vi "MICSD Do CCA.vi"(8 "error in (no error)":errorcluster, 9 "Use Averaging?":bool=TRUE, 10 "RSSI Mode":u8, 11 "VISA Resource Name":refnum<visa-resource-name>) -> (0 "error out":errorcluster, 1 "CCA Data":u16[](array[numeric]) format="%04x", 2 "Selected Channel":u8, 3 "dup VISA Resource Name":refnum<visa-resource-name>)   [LabVIEW 2020]
uses:
  <vilib>/Instr/_visa.llb/VISA Configure Serial Port (Instr).vi
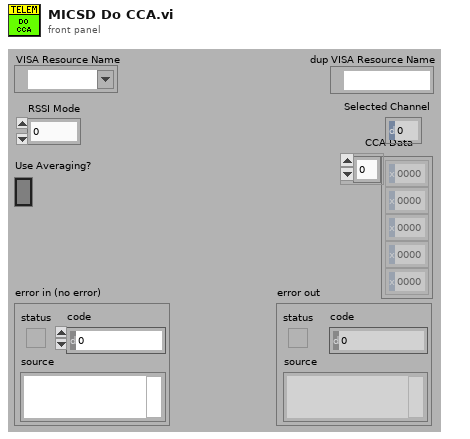
[diagram p1: front panel]
types:
  T1 = cluster{"Command Token":u8, "Length":u16, "Pack Data":u8[]}
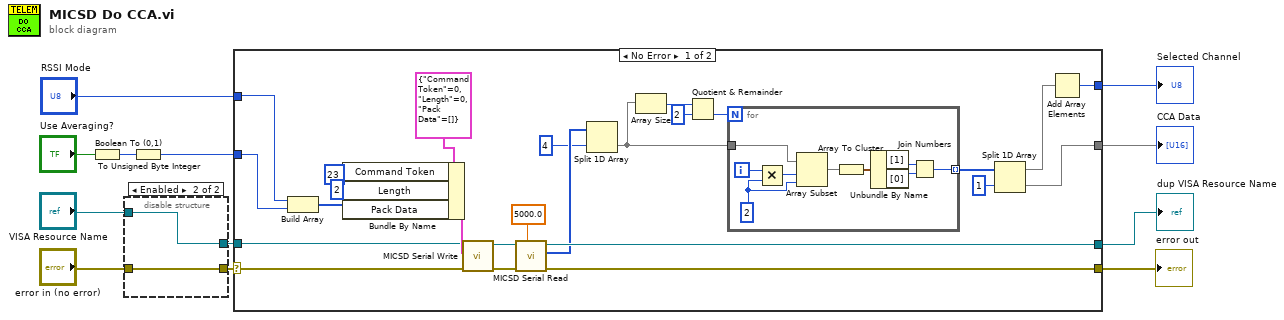
[diagram p0: block diagram]
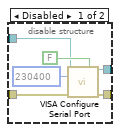
[diagram p2: hidden frame]
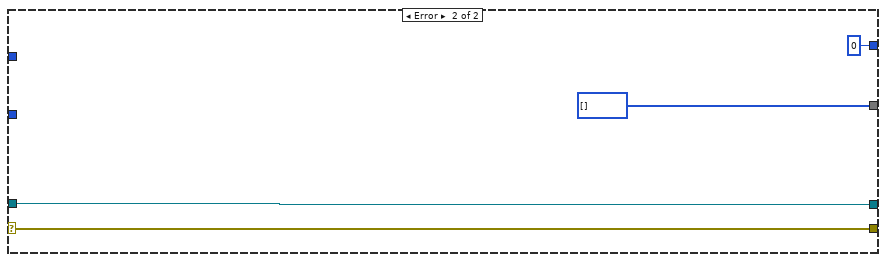
[diagram p3: hidden frame]
diagram:
  n1 = Boolean To (0,1)(Boolean="Use Averaging?") -> (0, 1=w3:i16)
  n2 = disable-structure shown="Enabled" {
    disable-tunnel: [w16 w19] -> w12
    disable-tunnel: [w15 w20] -> w11
    disable-tunnel: "VISA Resource Name" -> [w14 w20]
    disable-tunnel: "error in (no error)" -> [w13 w19]
    frame Disabled {
      n3 = call-poly "VISA Configure Serial Port"("VISA resource name"=w14, "Enable Termination\nChar (T)"=FALSE ("Enable Termination\nChar (T)"), "baud rate (9600)"=u32 230400, "error in (no error)"=w13) -> ("VISA resource name out"=w15:refnum<visa-resource-name>, "error out"=w16:errorcluster)  [unwired: 10 in]
    }
    frame Enabled {
    }
  }
  n4 = To Unsigned Byte Integer(number=w3) -> (unsigned 8bit integer=w2:u8)
  n5 = case shown="No Error" w12 {
    selector: w12 -> [w33 w58]
    tunnel: [w40 w58] -> w7
    tunnel: w11 -> [w34 w57]
    tunnel: [w39 w57] -> w8
    tunnel: [w24 u8[] []] -> w6
    tunnel: "RSSI Mode" -> [w31 _]
    tunnel: w2 -> [w30 _]
    tunnel: [w22 u16 0] -> w1
    frame No Error {
      n6 = Build Array(w31, w30) -> (w32:u8[])
      n7 = Bundle By Name(cluster=T1 {"Command Token"=0, "Length"=0, "Pack Data"=[]} ("Write Data"), "Command Token"=u8 23, "Length"=u16 2, "Pack Data"=w32) -> (w45:T1)
      n8 = call "MICSD Serial Write.vi"("error in (no error)"=w33, "Write Data"=w45, "VISA Resource Name"=w34) -> ("error out"=w38:errorcluster, "DUP Visa Resource Name"=w43:refnum<visa-resource-name>)  [unwired: 7 in]
      n9 = call "MICSD Serial Read.vi"("Timeout(mS)"=5000.0, "error in (no error)"=w38, "VISA Resource Name"=w43) -> ("error out"=w40:errorcluster, "Read Data"=w37:u8[], "DUP Visa Resource Name"=w39:refnum<visa-resource-name>)  [unwired: 6 in]
      n10 = Split 1D Array(array=w37, index=4) -> (second subarray=w29:u8[])  [unwired: 1 out]
      n11 = Array Size(array=w29) -> (size(s)=w28:i32)
      n12 = Quotient & Remainder(x=w28, y=2) -> (floor(x/y)=w27:i32)  [unwired: 1 out]
      n13 = for {
        N: w27 -> [_]
        tunnel: w29 -> [w51]
        tunnel: [w46] -> w25 mode=indexing
        i -> [w54]
        w52 = 2 ("y")
        n14 = Multiply(x=w54, y=w52) -> (x*y=w53:i32)
        n15 = Array Subset(array=w51, index=w53, length=w52) -> (w50:u8[])
        n16 = Array To Cluster(array=w50) -> (cluster=w49:cluster{"[0]":u8, "[1]":u8})
        n17 = Unbundle By Name(w49) -> ("[1]"=w48:u8, "[0]"=w47:u8)
        n18 = Join Numbers(hi=w48, lo=w47) -> ((hi.lo)=w46:u16)
      }
      n19 = Split 1D Array(array=w25, index=1) -> (first subarray=w21:u16[], second subarray=w24:u16[])
      n20 = Add Array Elements(numeric array=w21) -> (sum=w22:u16)
    }
    frame Error {
    }
  }
  "dup VISA Resource Name" <- w8
  "error out" <- w7
  "CCA Data" <- w6
  "Selected Channel" <- w1
